vi "graph_temperature.vi"() -> ()   [LabVIEW 2021]
uses:
  <vilib>/Analysis/1siggen.llb/Ramp Pattern by Delta.vi
  <vilib>/Analysis/NI_AALBase.lvlib
panel:
  out "Curva de temperatura":cluster{"Ramp Pattern":dbl[], u32[]}(graph)
  out "Array":string[](array[string])
  in  "file path (dialog if empty)":path
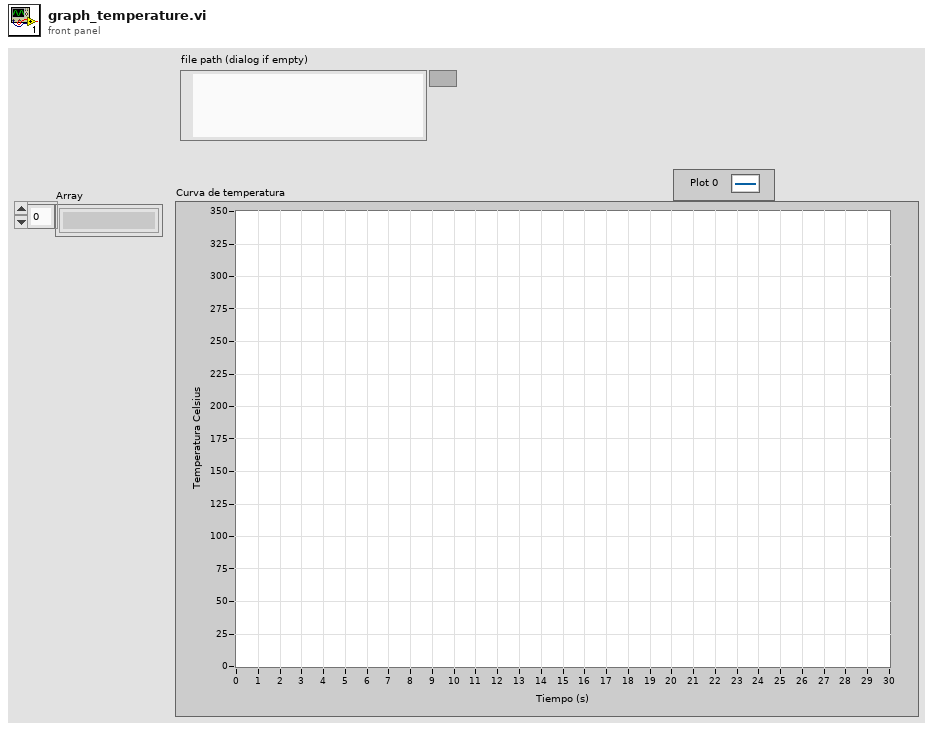
[diagram p1: front panel]
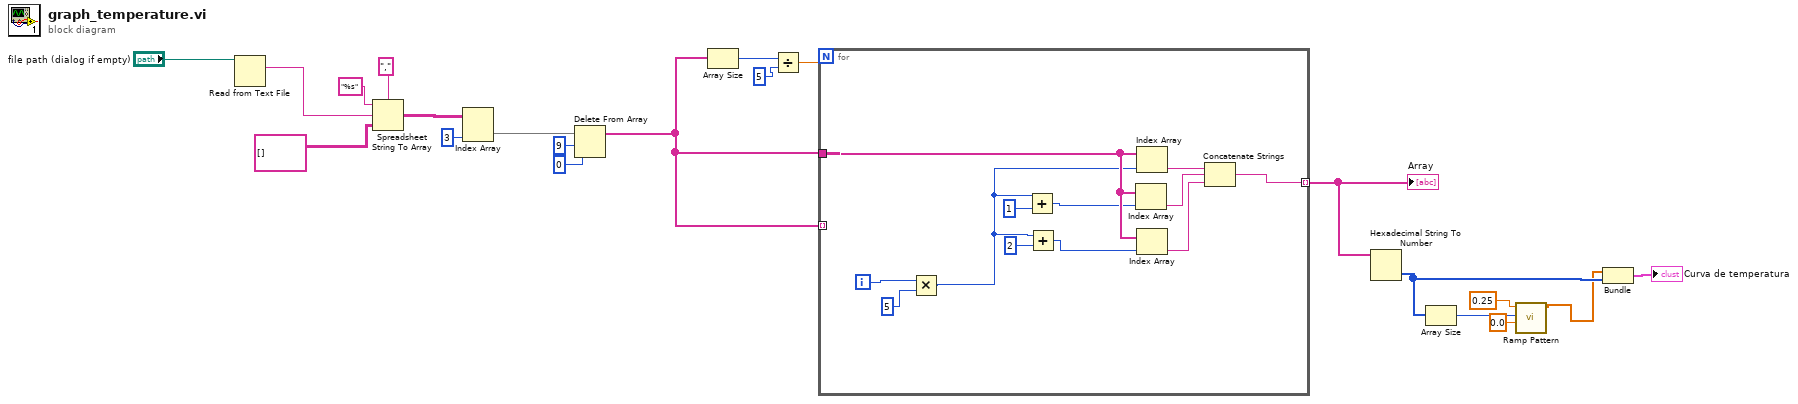
[diagram p0: block diagram]
diagram:
  n1 = Read from Text File(file (use dialog)="file path (dialog if empty)") -> (text=w19:string)  [unwired: 3 in, 3 out]
  n2 = Spreadsheet String To Array(delimiter (Tab)=",", format string="%s", spreadsheet string=w19, array type (2D Dbl)=string[][] [] ("Array")) -> (array=w16:string[][])
  n3 = Index Array(array=w16, index (col)=3 ("disabled index (col)")) -> (element=w14:string[])  [unwired: 1 in]
  n4 = Delete From Array(array=w14, length=9, index=0) -> (array with subset deleted=w11:string[])  [unwired: 1 out]
  n5 = Array Size(array=w11) -> (size(s)=w10:i32)
  n6 = Divide(x=w10, y=5) -> (x/y=w8:dbl)
  n7 = for {
    N: w8 -> [_]
    tunnel: w11 -> [_] mode=indexing
    tunnel: w11 -> [w33]
    tunnel: [w29] -> w7 mode=indexing
    i -> [w24]
    n8 = Multiply(x=w24, y=5) -> (x*y=w22:i32)
    n9 = Add(x=w22, y=1) -> (x+y=w26:i32)
    n10 = Add(x=w22, y=2) -> (x+y=w25:i32)
    n11 = Index Array(array=w33, index=w26) -> (element=w31:string)
    n12 = Index Array(array=w33, index=w22) -> (element=w32:string)
    n13 = Index Array(array=w33, index=w25) -> (element=w30:string)
    n14 = Concatenate Strings(w32, w31, w30) -> (w29:string)
  }
  "Array" <- w7
  n15 = Hexadecimal String To Number(string=w7) -> (number=w3:u32[])  [unwired: 2 in, 1 out]
  n16 = Array Size(array=w3) -> (size(s)=w6:i32)
  n17 = call-poly <vilib>:"Ramp Pattern.vi"("start"=0.0, "end"=w6, "delta"=0.25) -> ("Ramp Pattern"=w2:dbl[])  [unwired: 6 in, 2 out]
  n18 = Bundle("Ramp Pattern"=w2, w3) -> (→"Curva de temperatura":cluster{"Ramp Pattern":dbl[], u32[]})  [unwired: 1 in]
